vi "ConvertStringtoROS.vi"(1 "string in":string) -> (0 "ROS":T1={"topic port"=0, "Node"="", "topic"="", "type"="", "node port"=0, "error "={"status"=FALSE, "code"=0, "source"=""}, "Direction"=enum."Node", "Update (ms)"=1, "FIFO size"=1})   [LabVIEW 2015]
doc: "Unflatten a string using the ROS typdef. This is used when sending ROS settings with a queue."
uses:
  _ROSControl.ctl
  _ROSDirection.ctl
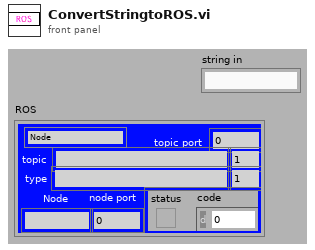
[diagram p1: front panel]
types:
  T1 = typedef "_ROSControl.ctl" = cluster{"topic port":u16, "Node":string, "topic":string, "type":string, "node port":u16, "error ":errorcluster, "Direction":T2, "Update (ms)":u16, "FIFO size":u16}
  T2 = typedef "_ROSDirection.ctl" = enum16{"Node", "Publisher", "Subscriber", "ServiceClient", "ServiceProvider"}
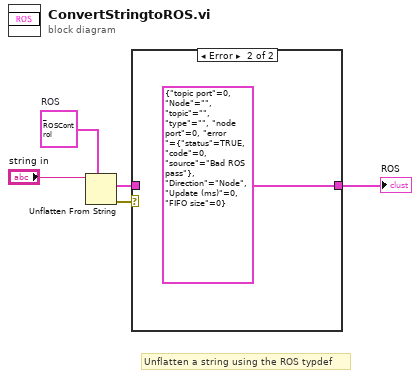
[diagram p0: block diagram]
diagram:
  w4 = T1 {"topic port"=0, "Node"="", "topic"="", "type"="", "node port"=0, "error "={"status"=FALSE, "code"=0, "source"=""}, "Direction"=enum."Node", "Update (ms)"=0, "FIFO size"=0}  # ROS
  # "Unflatten a string using the ROS typdef"
  n1 = Unflatten From String(type=w4, binary string="string in") -> (value=w1:T1, error out=w3:errorcluster)  [unwired: 3 in, 1 out]
  n2 = case shown="Error" w3 {
    tunnel: [w6 T1 {"topic port"=0, "Node"="", "topic"="", "type"="", "node port"=0, "error "={"status"=TRUE, "code"=0, "source"="Bad ROS pass"}, "Direction"=enum."Node", "Update (ms)"=0, "FIFO size"=0} ("ROS")] -> w2
    tunnel: w1 -> [w6 _]
    frame No Error {
    }
    frame Error {
    }
  }
  "ROS" <- w2
